vi "PID Fuzzy Control.vi"() -> ()   [LabVIEW 2019]
uses:
  <vilib>/rvi/interface/nirviMethod/nirviMethod.xnode
  <vilib>/FPGAPlugInAG/Dynamic/niLvFpga_Abort_Dynamic.vi
  <vilib>/FPGAPlugInAG/Dynamic/niLvFpga_Run_Dynamic.vi
  <vilib>/rvi/interface/nirviReadWriteControl/nirviReadWriteControl.xnode
  NiFpgaLv.dll
  <vilib>/Utility/error.llb/Error Cluster From Error Code.vi
  <vilib>/rvi/interface/Simulation/niFpgaSimulationCallBeginRW.vi
  <vilib>/rvi/errors/niLvFpgaAdjustHostInterfaceError.vi
  <vilib>/Platform/TimedLoop/XDataNode/wakeup.ctl
  <vilib>/Platform/TimedLoop/XDataNode/XDNodeRunTimeDep.lvlib
  <vilib>/Platform/TimedLoop/XDataNode/nitl_modes.ctl
  <vilib>/Platform/TimedLoop/XDataNode/timing_clust.ctl
  <vilib>/platform/TimedLoop/XDataNode/XDataNode.xnode
  <vilib>/addons/control/pid/NI_PID_pid.lvlib
  <vilib>/addons/control/pid/pid.llb/PID (DBL).vi
  <vilib>/Instr/_visa.llb/VISA Configure Serial Port (Instr).vi
  <vilib>/rvi/interface/nirviOpenFPGA/nirviOpenFPGA.xnode
  <vilib>/addons/Fuzzy Logic/NI_Fuzzy_Logic_API.lvlib
  <vilib>/addons/Fuzzy Logic/FL Fuzzy Controller (SISO).vi
panel:
  out "Numeric":i32
  out "L1 P補償值":dbl
  out "L2 P補償值":dbl
  out "L3 P補償值":dbl
  out "L1 誤差":dbl
  out "L2 誤差":dbl
  out "L3 誤差":dbl
  out "目標角度Chart":cluster{dbl, dbl}[](graph) caption="Waveform Chart - dark"
  in  "VISA resource name":refnum<visa-resource-name>="COM2"
  out "Axis 3比較":cluster{i32[], dbl[]}[](graph)
  out "Axis 2比較":cluster{i32[], dbl[]}[](graph)
  out "Axis 1比較":cluster{i32[], dbl[]}[](graph)
  out "Axis 1":cluster{i32[], dbl[]}(graph)
  out "Axis 3":cluster{i32[], dbl[]}(graph)
  out "Axis 2":cluster{i32[], dbl[]}(graph)
  in  "Period":i64=10
  in  "stop":bool
  out "time loop error":errorcluster
  out "Axis 1 速率 (1mm/s)":dbl
  out "Real Period":u32
  out "沖壓":bool
  out "結束了":bool
  out "Voltage\nOutput":dbl
  out "Voltage\nOutput 2":dbl
  out "Voltage\nOutput 3":dbl
  out "Axis 2 速率 (1mm/s)":dbl
  out "Axis 3 速率 (1mm/s)":dbl
  in  "Axis1 PID gains":T1={"proportional gain (Kc)"=2.0, "integral time (Ti, min)"=0.0, "derivative time (Td, min)"=0.0} {"derivative time (Td, min)" format="%.3f"; "integral time (Ti, min)" format="%.3f"; "proportional gain (Kc)" format="%.3f"}
  in  "Axis 2 PID gains":T1={"proportional gain (Kc)"=2.0, "integral time (Ti, min)"=0.0, "derivative time (Td, min)"=0.0} {"derivative time (Td, min)" format="%.3f"; "integral time (Ti, min)" format="%.3f"; "proportional gain (Kc)" format="%.3f"}
  in  "Axis 3 PID gains":T1={"proportional gain (Kc)"=2.0, "integral time (Ti, min)"=0.0, "derivative time (Td, min)"=0.0} {"derivative time (Td, min)" format="%.3f"; "integral time (Ti, min)" format="%.3f"; "proportional gain (Kc)" format="%.3f"}
  out "實際角度":cluster{"A":dbl, "B":dbl}={"A"=-3.299667554384925, "B"=3.520332445615068}
  out "陀螺儀推算軸長L1":dbl
  out "陀螺儀推算軸長L2":dbl
  out "陀螺儀推算軸長L3":dbl
  out "目標軸長L1":dbl
  out "目標軸長L2":dbl
  out "目標軸長L3":dbl
  out "實際角度Chart":cluster{"X":dbl, "Y":dbl}(graph)={"X"=-3.299667554384925, "Y"=3.520332445615068} caption="Waveform Chart - dark"
  out "目標A":dbl
  out "目標B":dbl
  out "shutdown error":errorcluster
  in  "Tab Control":enum32{"Axis Control"}(tab)
  in  "Axis 1~3 Servo on?":bool
  out "Axis 3 Backward Limit":bool
  out "Axis 3 Backward Limit 2":bool
  out "Axis 2 Backward Limit":bool
  out "Axis 2 Backward Limit 2":bool
  in  "Axis 3 Alarm Reset":bool
  in  "Axis 2 Alarm Reset":bool
  in  "Axis 3 Position Reset":bool
  in  "Axis 2 Position Reset":bool
  in  "Axis 1 Alarm Reset":bool
  in  "Axis 1 Position Reset":bool
  in  "Axis 3 Speed":fxp<+/-,64,32>
  in  "Axis 2 Speed":fxp<+/-,64,32>
  out "Axis 3 Encoder Position (Counts)":i32
  out "Axis 2 Encoder Position (Counts)":i32
  out "Axis 1 Encoder Position (Counts)":i32
  in  "Axis 1 Spped":fxp<+/-,64,32>
  in  "Axis 2 Servo on?":bool
  in  "Axis 3 Servo on?":bool
  in  "Axis 1 Servo on?":bool
  out "Axis 1 Forward Limit":bool
  out "Axis 1 Backward Limit":bool
  out "Timed Out?":bool
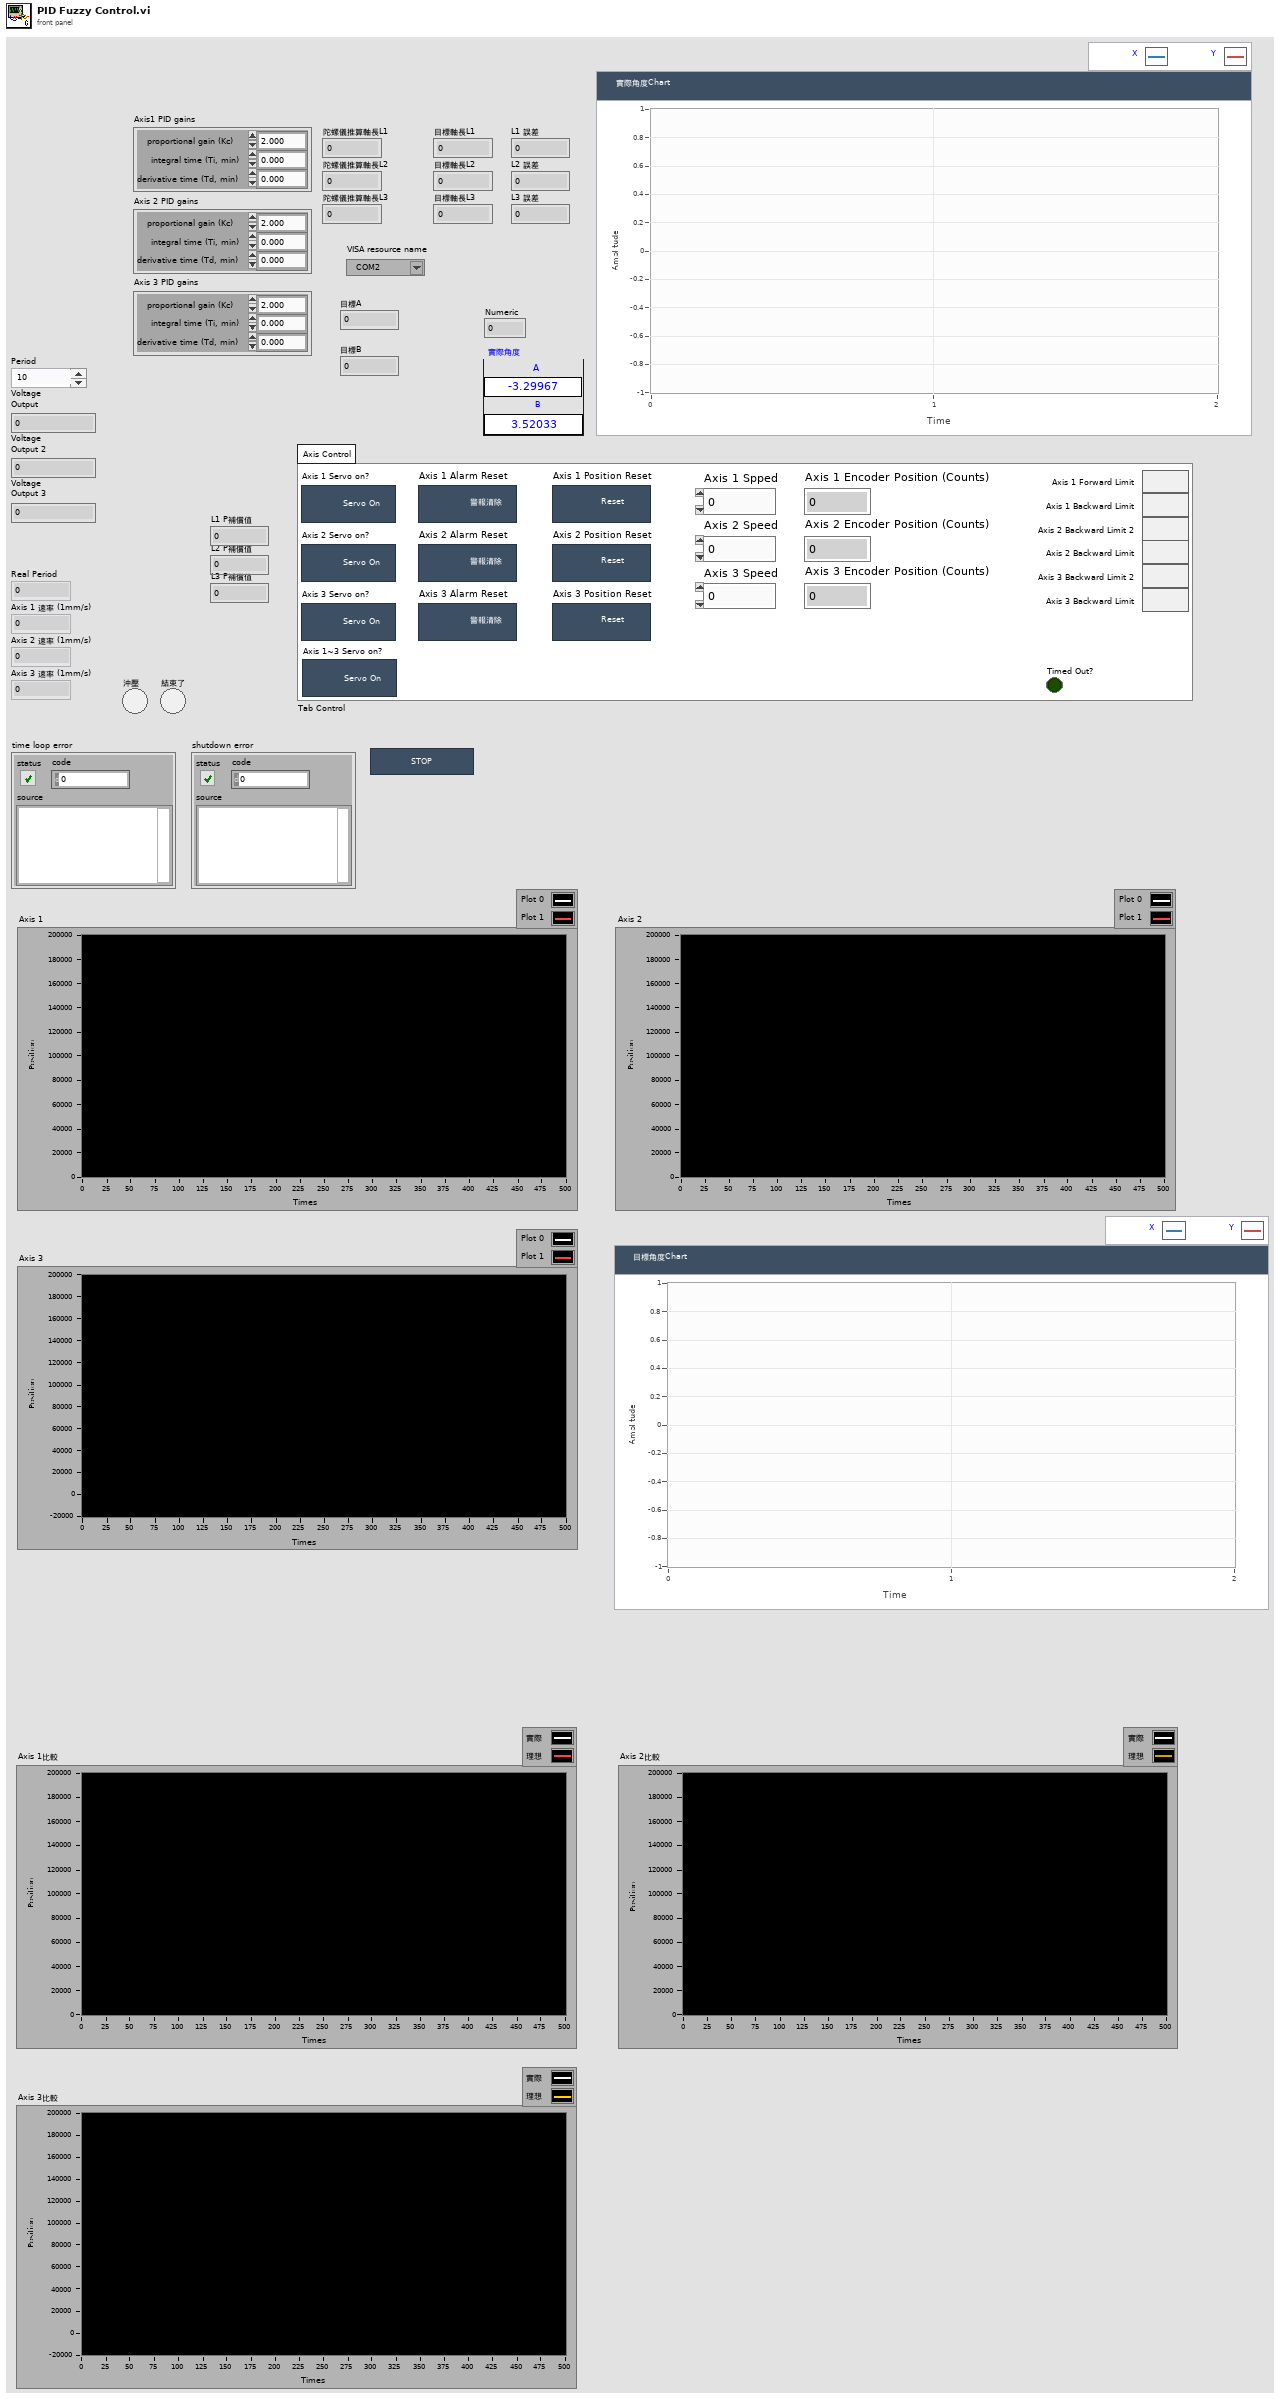
[diagram p1: front panel]
types:
  T1 = cluster{"proportional gain (Kc)":dbl, "integral time (Ti, min)":dbl, "derivative time (Td, min)":dbl}
  T2 = enum16{"open", "replace", "create", "open or create", "replace or create", "replace or create with confirmation"}
  T3 = typedef "XDNodeRunTimeDep.lvlib/timing_clust.ctl" = cluster{"Expected End [f-1]":u64, "Actual End [f-1]":u64, "Finished Late? [f-1]":bool, "Expected End [i-1]":u64, "Actual End [i-1]":u64, "Finished Late? [i-1]":bool, "Expected Start [i]":u64, "Actual Start [i]":u64, "Expected Start [f]":u64, "Actual Start [f]":u64, "Source Name":string, "Structure Name":string, "Period":i64, "Deadline":i64, "Offset":i64, "Start":i64, "Priority":i32, "Timeout":i32, "Mode":T4, "Wakeup Reason":T5, "Error":errorcluster, "Source Type":string, "Secondary Source Type":string, "Global End Time":u64, "Global Start Time":u64, "Frame Duration":u64, "Iteration Duration":u64, "Assigned CPU":i32, "I/O Scan Engine Mode":u32}
  T4 = typedef "XDNodeRunTimeDep.lvlib/nitl_modes.ctl" = enum32{"No Change", "Process missed periods, maintain original phase", "Discard missed periods, maintain original phase", "Process missed periods, ignore original phase", "Discard missed periods, ignore original phase"}
  T5 = typedef "XDNodeRunTimeDep.lvlib/wakeup.ctl" = enum32{"Normal", "Aborted", "Asynchronous wakeup", "Timing source error", "Timed loop error", "Timeout"}
  T6 = typedef "NI_Fuzzy_Logic_API.lvlib/FL System.ctl" = cluster{"input variables":T7[], "output variables":T7[], "rules":T10[], "defuzzification method":T16, "description":string, "user MF interpolating polynomials":T17[]}
  T7 = typedef "NI_Fuzzy_Logic_API.lvlib/FL Variable.ctl" = cluster{"name":string, "range":dbl[], "MFs":T8[]}
  T8 = typedef "NI_Fuzzy_Logic_API.lvlib/FL Membership Function.ctl" = cluster{"name":string, "shape":T9, "points":dbl[], "color":u32, "user-defined shape index":i32}
  T9 = typedef "NI_Fuzzy_Logic_API.lvlib/FL Membership Function Shape.ctl" = u16
  T10 = typedef "NI_Fuzzy_Logic_API.lvlib/FL Rule.ctl" = cluster{"antecedents":T11[], "antecedent connective":T13, "consequents":T14[], "consequent implication":T15, "degree of support":dbl}
  T11 = typedef "NI_Fuzzy_Logic_API.lvlib/FL Antecedent.ctl" = cluster{"Var Index":i32, "MF Index":i32, "Cond":T12}
  T12 = typedef "NI_Fuzzy_Logic_API.lvlib/FL Modifier.ctl" = u16
  T13 = typedef "NI_Fuzzy_Logic_API.lvlib/FL Antecedent Connective.ctl" = u16
  T14 = typedef "NI_Fuzzy_Logic_API.lvlib/FL Consequent.ctl" = cluster{"Var Index":i32, "MF Index":i32, "Cond":T12}
  T15 = typedef "NI_Fuzzy_Logic_API.lvlib/FL Consequent Implication.ctl" = u16
  T16 = typedef "NI_Fuzzy_Logic_API.lvlib/FL Defuzzification.ctl" = u16
  T17 = typedef "NI_Fuzzy_Logic_API.lvlib/FL Interpolating polynomials.ctl" = cluster{"X":dbl[], "Y":dbl[], "Y(x) coeff":dbl[][], "X(y) coeff":dbl[][], "Area(y) coeff":dbl[][], "coa_x(y) coeff":dbl[][]}
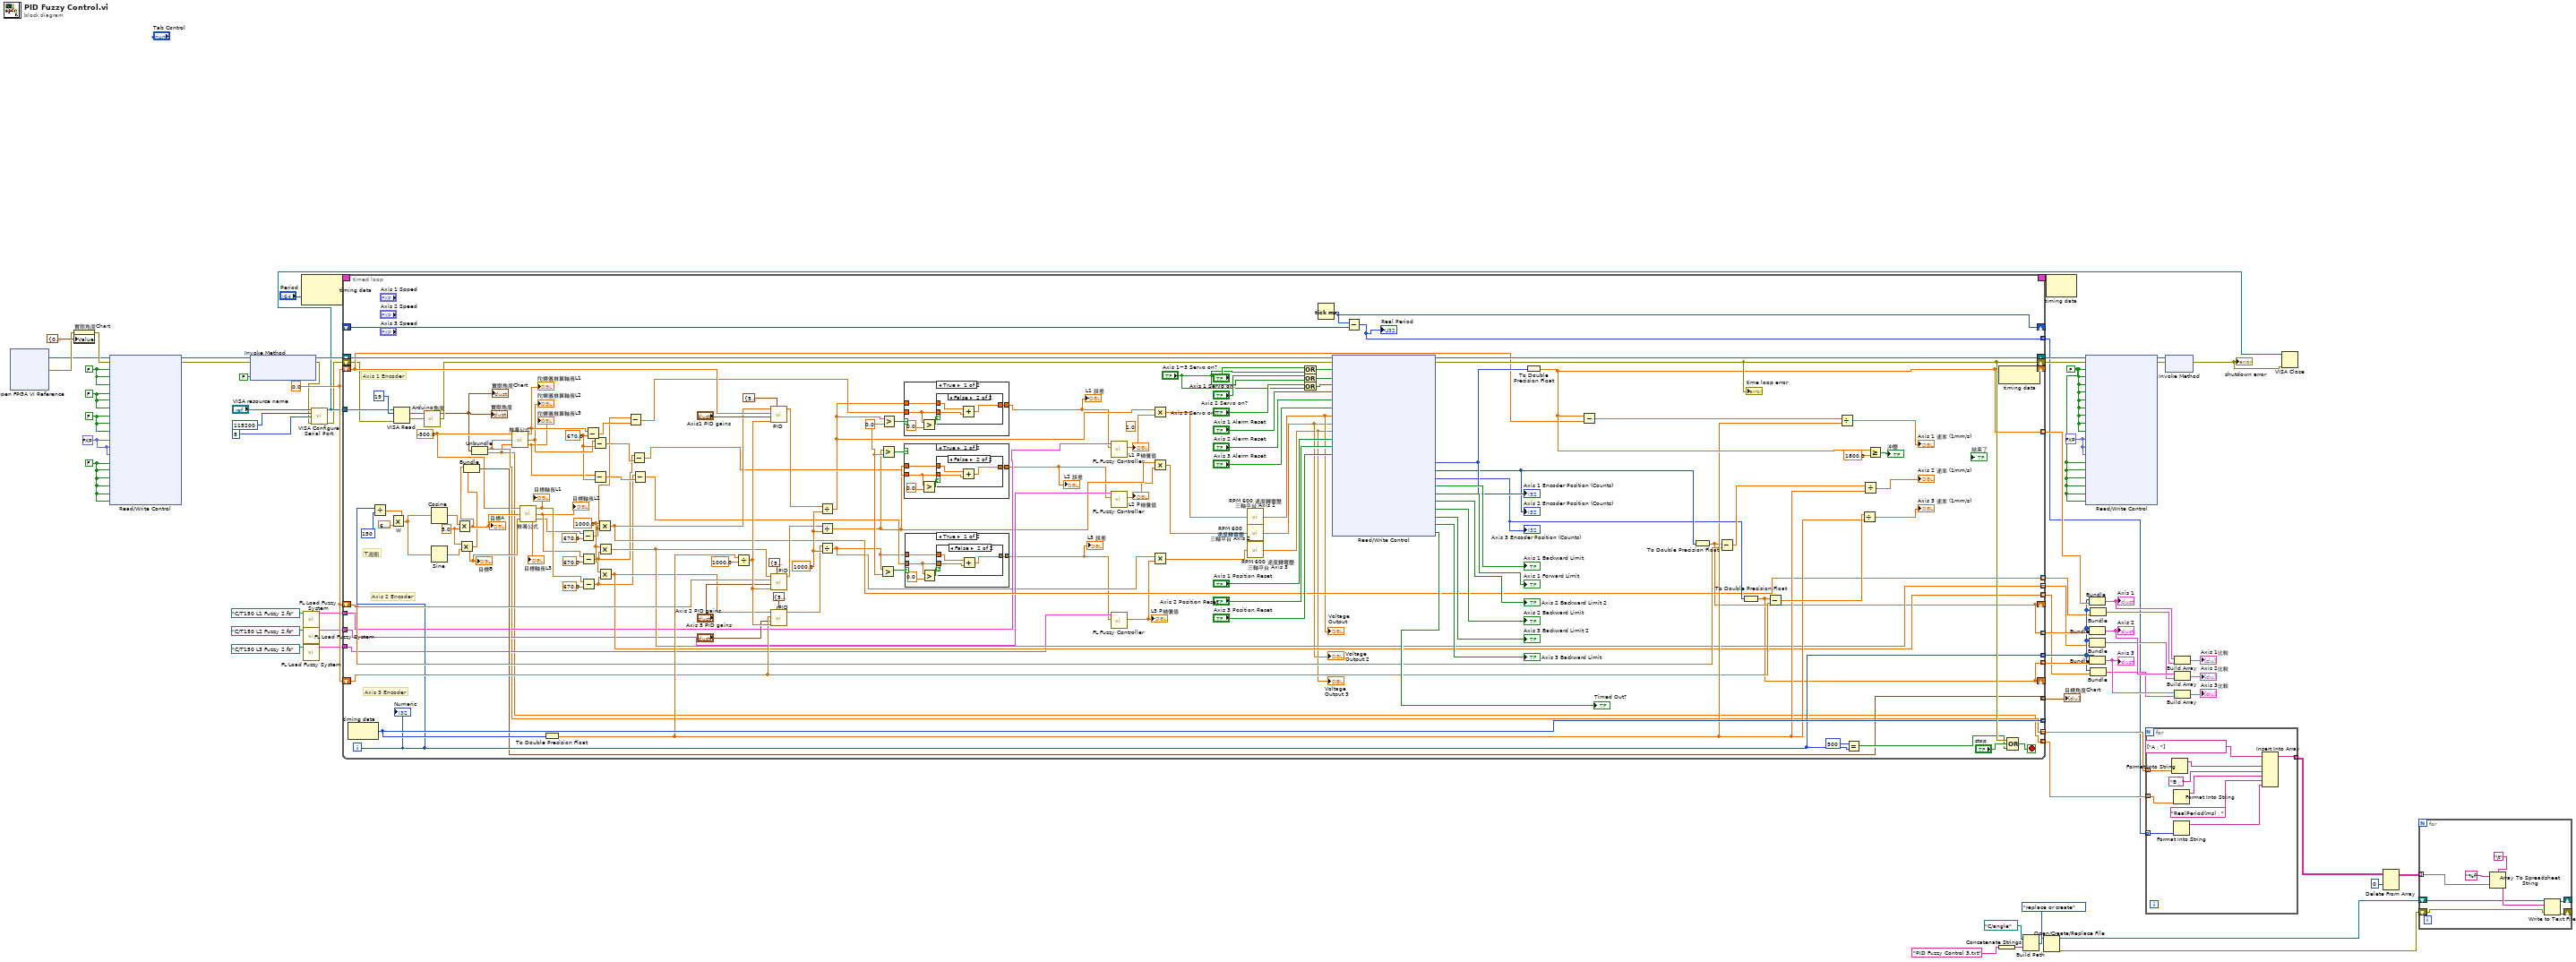
[diagram p0: block diagram]
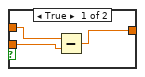
[diagram p2: hidden frame]
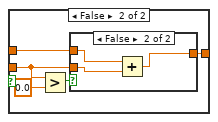
[diagram p3: hidden frame]
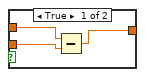
[diagram p4: hidden frame]
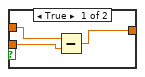
[diagram p5: hidden frame]
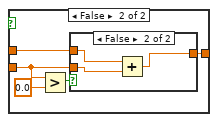
[diagram p6: hidden frame]
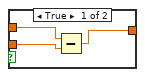
[diagram p7: hidden frame]
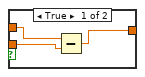
[diagram p8: hidden frame]
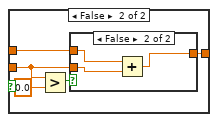
[diagram p9: hidden frame]
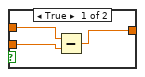
[diagram p10: hidden frame]
diagram:
  w25 = FALSE
  w27 = FALSE
  w52 = 0.0
  w31 = fxp<+,1,1> 0.0
  w30 = FALSE
  w28 = FALSE
  w26 = fxp<+,1,1> 0.0
  w29 = FALSE
  n1 = xnode "Open FPGA VI Reference"() -> ("FPGA VI Reference Out"=w23:refnum<k20>, "error out"=w24:errorcluster)  [unwired: 2 in]
  n2 = property on="實際角度Chart" class="WFChart (strict)"(error in=w24, "Value"=cluster{"X":dbl, "Y":dbl} {"X"=0.0, "Y"=0.0} ("實際角度Chart")) -> (error out=w33:errorcluster)  [unwired: 1 in, 1 out]
  n3 = xnode "Read/Write Control"("FPGA VI Reference In"=w23, "error in"=w33, "Axis 1 Servo on?"=w29, "Axis 2 Servo on?"=w29, "Axis 3 Servo on?"=w29, "Axis 1 Alarm Reset"=w28, "Axis 2 Alarm Reset"=w28, "Axis 3 Alarm Reset"=w28, "Axis 1 Position Reset"=w27, "Axis 2 Position Reset"=w27, "Axis 3 Position Reset"=w27, "Axis 1 Voltage In"=w26, "Axis 2 Voltage In"=w26, "Axis 3 Voltage In"=w26, "Axis 1 Backward Limit"=w25, "Axis 1 Forward Limit"=w25, "Axis 2 Forward Limit"=w25, "Axis 2 Backward Limit"=w25, "Axis 3 ForWard Limit"=w25, "Axis 3 Backward Limit"=w25) -> ("FPGA VI Reference Out"=w64:refnum<k20>, "error out"=w63:errorcluster)
  n4 = xnode "Invoke Method"("FPGA VI Reference In"=w64, "error in"=w63, "Wait Until Done (F)"=FALSE) -> ("FPGA VI Reference Out"=w61:refnum<k20>, "error out"=w22:errorcluster)
  n5 = node-c288("Period") -> (w66:T3)  [unwired: 1 in]
  n6 = call <vilib>:"FL Load Fuzzy System.vi"("file path"=path "C:/T150 L1 Fuzzy 2.fs") -> ("fuzzy system out"=w16:T6)  [unwired: 9 in, 1 out]
  n7 = call <vilib>:"FL Load Fuzzy System.vi"("file path"=path "C:/T150 L2 Fuzzy 2.fs") -> ("fuzzy system out"=w15:T6)  [unwired: 9 in, 1 out]
  n8 = call <vilib>:"FL Load Fuzzy System.vi"("file path"=path "C:/T150 L3 Fuzzy 2.fs") -> ("fuzzy system out"=w14:T6)  [unwired: 9 in, 1 out]
  n9 = call-poly "VISA Configure Serial Port"("VISA resource name"="VISA resource name", "baud rate (9600)"=u32 115200, "data bits (8)"=u16 8, "error in (no error)"=w22) -> ("VISA resource name out"=w40:refnum<visa-resource-name>, "error out"=w21:errorcluster)  [unwired: 10 in]
  n10 = timed-loop {
    shift-right: [w192] -> w57
    shift-left: w61 -> [w191]
    shift-right: [w159] -> w58
    shift-left: w21 -> [w124]
    timing: w66 -> [_]
    timing-out: [_] -> w65
    shift-right: [w154] -> _
    shift-left: w52 -> [w153]
    tunnel: [w158] -> _ mode=indexing
    shift-right: [w188] -> _
    shift-left: _ -> [w189]
    tunnel: [w121] -> w1 mode=indexing
    shift-right: [w113] -> _
    shift-left: w52 -> [w148]
    shift-right: [w112] -> _
    shift-left: w52 -> [w149]
    tunnel: [w129] -> w51 mode=indexing
    tunnel: [w154] -> w55 mode=indexing
    tunnel: [w113] -> w54 mode=indexing
    tunnel: [w112] -> w53 mode=indexing
    tunnel: w40 -> [w125]
    tunnel: [w116] -> w39 mode=indexing
    tunnel: [w115] -> w38 mode=indexing
    tunnel: [w114] -> w37 mode=indexing
    tunnel: [w106] -> w20 mode=indexing
    tunnel: w16 -> [w92]
    tunnel: w15 -> [w91]
    tunnel: w14 -> [w90]
    tunnel: [w82] -> w3 mode=indexing
    tunnel: [w81] -> w2 mode=indexing
    i -> [w129]
    stop <- w190 stop-if-true
    (unwired) 1.0
    w95 = 670.0 ("y")
    w103 = 0.0 ("y")
    w120 = 1000.0 ("x")
    w138 = 5.0 ("y")
    w98 = -500.0 ("移動z")
    w128 = 1000.0 ("x")
    # "T週期"
    # "Axis 3 Encoder"
    # "Axis 2 Encoder"
    # "Axis 1 Encoder"
    n11 = node-c288() -> (w158:i64)  [unwired: 1 in]
    n12 = Divide(x=w129, y=150) -> (x/y=w134:dbl)
    n13 = Multiply "W"(x=w134, y=6.283185307179586) -> (x*y=w133:dbl)
    n14 = VISA Read(VISA resource name=w125, byte count=u32 19, error in (no error)=w124) -> (read buffer=w122:string, error out=w126:errorcluster)  [unwired: 2 out]
    n15 = call "Arduino角度.vi"("error in"=w126, "read buffer"=w122) -> ("error out"=w123:errorcluster, "Waveform Chart"=w70:cluster{dbl, dbl})  [unwired: 1 in, 1 out]
    "實際角度" <- w70
    "實際角度Chart" <- w70
    n16 = Cosine(x=w133) -> (cos(x)=w135:dbl)
    n17 = Sine(x=w133) -> (sin(x)=w136:dbl)
    n18 = Multiply(x=w135, y=w138) -> (x*y=w108:dbl)
    "目標A" <- w108
    n19 = Multiply(x=w138, y=w136) -> (x*y=w107:dbl)
    "目標B" <- w107
    n20 = Bundle(w108, w107) -> (w106:cluster{dbl, dbl})  [unwired: 1 in]
    n21 = Unbundle(w70) -> (w82:dbl, w81:dbl)
    n22 = call "推導公式.vi"("be"=w81, "al"=w82, "移動z"=w98) -> ("L3"=w80:dbl, "L2"=w96:dbl, "L1"=w97:dbl)
    "陀螺儀推算軸長L1" <- w97
    "陀螺儀推算軸長L2" <- w96
    "陀螺儀推算軸長L3" <- w80
    n23 = call "推導公式.vi"("be"=w107, "al"=w108, "移動z"=w98) -> ("L3"=w99:dbl, "L2"=w100:dbl, "L1"=w101:dbl)
    "目標軸長L1" <- w101
    "目標軸長L2" <- w100
    "目標軸長L3" <- w99
    n24 = To Double Precision Float(number=w158) -> (double precision float=w151:dbl)
    n25 = Subtract(x=w99, y=670.0) -> (x-y=w83:dbl)
    n26 = Subtract(x=w100, y=670.0) -> (x-y=w85:dbl)
    n27 = Subtract(x=w101, y=670.0) -> (x-y=w88:dbl)
    n28 = Subtract(x=w97, y=w95) -> (x-y=w93:dbl)
    n29 = Subtract(x=w96, y=w95) -> (x-y=w86:dbl)
    n30 = Subtract(x=w80, y=w95) -> (x-y=w94:dbl)
    n31 = Multiply(x=w128, y=w83) -> (x*y=w116:dbl)
    n32 = Multiply(x=w128, y=w85) -> (x*y=w115:dbl)
    n33 = Multiply(x=w128, y=w88) -> (x*y=w114:dbl)
    n34 = Subtract(x=w83, y=w93) -> (x-y=w84:dbl)
    n35 = Subtract(x=w85, y=w86) -> (x-y=w87:dbl)
    n36 = Subtract(x=w88, y=w94) -> (x-y=w89:dbl)
    n37 = Divide(x=w151, y=1000.0) -> (x/y=w150:dbl)
    n38 = call-poly <vilib>:"PID.vi"("output range"=cluster{"output high":dbl, "output low":dbl} {"output high"=50000.0, "output low"=-50000.0}, "dt (s)"=w150, "PID gains"="Axis1 PID gains", "process variable"=w153, "setpoint"=w116) -> ("output"=w119:dbl)  [unwired: 5 in, 1 out]
    n39 = call-poly <vilib>:"PID.vi"("output range"=cluster{"output high":dbl, "output low":dbl} {"output high"=50000.0, "output low"=-50000.0}, "dt (s)"=w150, "PID gains"="Axis 2 PID gains", "process variable"=w148, "setpoint"=w115) -> ("output"=w118:dbl)  [unwired: 5 in, 1 out]
    n40 = call-poly <vilib>:"PID.vi"("output range"=cluster{"output high":dbl, "output low":dbl} {"output high"=50000.0, "output low"=-50000.0}, "dt (s)"=w150, "PID gains"="Axis 3 PID gains", "process variable"=w149, "setpoint"=w114) -> ("output"=w117:dbl)  [unwired: 5 in, 1 out]
    n41 = Divide(x=w119, y=w120) -> (x/y=w76:dbl)
    n42 = Divide(x=w118, y=w120) -> (x/y=w74:dbl)
    n43 = Divide(x=w117, y=w120) -> (x/y=w79:dbl)
    n44 = Greater?(x=w79, y=w103) -> (0:w102:bool)
    n45 = Greater?(x=w74, y=w103) -> (0:w104:bool)
    n46 = Greater?(x=w76, y=w103) -> (0:w105:bool)
    n47 = case shown="True" w105 {
      tunnel: [w240 w251] -> w73
      tunnel: w84 -> [w238 w249]
      tunnel: w76 -> [w239 w250]
      frame True {
        n48 = Greater?(x=w238, y=0.0) -> (0:w241:bool)
        n49 = case shown="False" w241 {
          tunnel: [w245 w248] -> w240
          tunnel: w239 -> [w244 w247]
          tunnel: w238 -> [w243 w246]
          frame True {
            n50 = Subtract(x=w244, y=w243) -> (x-y=w245:dbl)
          }
          frame False {
            n51 = Add(x=w247, y=w246) -> (x+y=w248:dbl)
          }
        }
      }
      frame False {
        n52 = Greater?(x=w249, y=0.0) -> (0:w252:bool)
        n53 = case shown="False" w252 {
          tunnel: [w256 w259] -> w251
          tunnel: w250 -> [w255 w258]
          tunnel: w249 -> [w254 w257]
          frame True {
            n54 = Subtract(x=w255, y=w254) -> (x-y=w256:dbl)
          }
          frame False {
            n55 = Add(x=w258, y=w257) -> (x+y=w259:dbl)
          }
        }
      }
    }
    "L1 誤差" <- w73
    n56 = case shown="True" w104 {
      tunnel: [w218 w229] -> w72
      tunnel: w87 -> [w216 w227]
      tunnel: w74 -> [w217 w228]
      frame True {
        n57 = Greater?(x=w216, y=0.0) -> (0:w219:bool)
        n58 = case shown="False" w219 {
          tunnel: [w223 w226] -> w218
          tunnel: w217 -> [w222 w225]
          tunnel: w216 -> [w221 w224]
          frame True {
            n59 = Subtract(x=w222, y=w221) -> (x-y=w223:dbl)
          }
          frame False {
            n60 = Add(x=w225, y=w224) -> (x+y=w226:dbl)
          }
        }
      }
      frame False {
        n61 = Greater?(x=w227, y=0.0) -> (0:w230:bool)
        n62 = case shown="False" w230 {
          tunnel: [w234 w237] -> w229
          tunnel: w228 -> [w233 w236]
          tunnel: w227 -> [w232 w235]
          frame True {
            n63 = Subtract(x=w233, y=w232) -> (x-y=w234:dbl)
          }
          frame False {
            n64 = Add(x=w236, y=w235) -> (x+y=w237:dbl)
          }
        }
      }
    }
    "L2 誤差" <- w72
    n65 = case shown="True" w102 {
      tunnel: [w196 w207] -> w71
      tunnel: w89 -> [w194 w205]
      tunnel: w79 -> [w195 w206]
      frame True {
        n66 = Greater?(x=w194, y=0.0) -> (0:w197:bool)
        n67 = case shown="False" w197 {
          tunnel: [w201 w204] -> w196
          tunnel: w195 -> [w200 w203]
          tunnel: w194 -> [w199 w202]
          frame True {
            n68 = Subtract(x=w200, y=w199) -> (x-y=w201:dbl)
          }
          frame False {
            n69 = Add(x=w203, y=w202) -> (x+y=w204:dbl)
          }
        }
      }
      frame False {
        n70 = Greater?(x=w205, y=0.0) -> (0:w208:bool)
        n71 = case shown="False" w208 {
          tunnel: [w212 w215] -> w207
          tunnel: w206 -> [w211 w214]
          tunnel: w205 -> [w210 w213]
          frame True {
            n72 = Subtract(x=w211, y=w210) -> (x-y=w212:dbl)
          }
          frame False {
            n73 = Add(x=w214, y=w213) -> (x+y=w215:dbl)
          }
        }
      }
    }
    "L3 誤差" <- w71
    n74 = call-poly <vilib>:"FL Fuzzy Controller.vi"("input value"=w73, "fuzzy system in"=w92) -> ("output value"=w69:dbl)  [unwired: 5 in, 4 out]
    "L1 P補償值" <- w69
    n75 = call-poly <vilib>:"FL Fuzzy Controller.vi"("input value"=w72, "fuzzy system in"=w91) -> ("output value"=w68:dbl)  [unwired: 5 in, 4 out]
    "L2 P補償值" <- w68
    n76 = call-poly <vilib>:"FL Fuzzy Controller.vi"("input value"=w71, "fuzzy system in"=w90) -> ("output value"=w67:dbl)  [unwired: 5 in, 4 out]
    "L3 P補償值" <- w67
    n77 = Multiply(x=w76, y=w69) -> (x*y=w75:dbl)
    n78 = Multiply(x=w74, y=w68) -> (x*y=w77:dbl)
    n79 = Multiply(x=w79, y=w67) -> (x*y=w78:dbl)
    n80 = call "RPM 600 速度轉電壓 三軸平台 Axis 1.vi"("Speed (1mm/s)"=w75) -> ("Voltage\nOutput"=w111:dbl)
    "Voltage\nOutput" <- w111
    n81 = call "RPM 600 速度轉電壓 三軸平台 Axis 2.vi"("Speed (1mm/s)"=w77) -> ("Voltage\nOutput"=w110:dbl)
    "Voltage\nOutput 2" <- w110
    n82 = call "RPM 600 速度轉電壓 三軸平台 Axis 3.vi"("Speed (1mm/s)"=w78) -> ("Voltage\nOutput"=w109:dbl)
    "Voltage\nOutput 3" <- w109
    n83 = Or(x="Axis 1 Servo on?", y="Axis 1~3 Servo on?") -> (x .or. y?=w171:bool)
    n84 = Or(x="Axis 2 Servo on?", y="Axis 1~3 Servo on?") -> (x .or. y?=w168:bool)
    n85 = Or(x="Axis 3 Servo on?", y="Axis 1~3 Servo on?") -> (x .or. y?=w166:bool)
    n86 = Tick Count (ms)() -> (millisecond timer value=w188:u32)
    n87 = xnode "Read/Write Control"("FPGA VI Reference In"=w191, "error in"=w123, "Axis 1 Servo on?"=w171, "Axis 2 Servo on?"=w168, "Axis 3 Servo on?"=w166, "Axis 1 Alarm Reset"="Axis 1 Alarm Reset", "Axis 2 Alarm Reset"="Axis 2 Alarm Reset", "Axis 3 Alarm Reset"="Axis 3 Alarm Reset", "Axis 1 Voltage In"=w111, "Axis 2 Voltage In"=w110, "Axis 3 Voltage In"=w109, "Axis 1 Position Reset"="Axis 1 Position Reset", "Axis 2 Position Reset"="Axis 2 Position Reset", "Axis 3 Position Reset"="Axis 3 Position Reset") -> ("FPGA VI Reference Out"=w192:refnum<k20>, "error out"=w159:errorcluster, "Axis 1 Encoder Position (Counts)"=w164:i32, "Axis 2 Encoder Position (Counts)"=w162:i32, "Axis 3 Encoder Position (Counts)"=w161:i32, "Axis 1 Backward Limit"=→"Axis 1 Backward Limit":bool, "Axis 1 Forward Limit"=→"Axis 1 Forward Limit":bool, "Axis 2 Backward Limit"=→"Axis 2 Backward Limit 2":bool, "Axis 2 Forward Limit"=→"Axis 2 Backward Limit":bool, "Axis 3 Backward Limit"=→"Axis 3 Backward Limit 2":bool, "Axis 3 ForWard Limit"=→"Axis 3 Backward Limit":bool, "Timed Out?"=→"Timed Out?":bool)
    "time loop error" <- w159
    "Axis 1 Encoder Position (Counts)" <- w164
    "Axis 2 Encoder Position (Counts)" <- w162
    "Axis 3 Encoder Position (Counts)" <- w161
    n88 = Subtract(x=w188, y=w189) -> (x-y=w121:u32)
    "Real Period" <- w121
    n89 = To Double Precision Float(number=w164) -> (double precision float=w154:dbl)
    n90 = Subtract(x=w154, y=w153) -> (x-y=w193:dbl)
    n91 = To Double Precision Float(number=w162) -> (double precision float=w113:dbl)
    n92 = Subtract(x=w113, y=w148) -> (x-y=w163:dbl)
    n93 = To Double Precision Float(number=w161) -> (double precision float=w112:dbl)
    n94 = Subtract(x=w112, y=w149) -> (x-y=w160:dbl)
    n95 = Divide(x=w193, y=w151) -> (x/y=→"Axis 1 速率 (1mm/s)":dbl)
    n96 = Equal?(x=500, y=w129) -> (x = y?=w140:bool)
    n97 = Divide(x=w160, y=w151) -> (x/y=→"Axis 3 速率 (1mm/s)":dbl)
    n98 = Divide(x=w163, y=w151) -> (x/y=→"Axis 2 速率 (1mm/s)":dbl)
    n99 = Greater Or Equal?(x=w154, y=1800.0) -> (x >= y?=→"沖壓":bool)
    n100 = node-c288() -> ()  [unwired: 1 in, 1 out]
    n101 = Compound Arithmetic op=OR(w159, "stop", w140) -> (w190:bool)
    "Numeric" <- w129
  }
  "目標角度Chart" <- w20
  n102 = Concatenate Strings("PID Fuzzy Control 3.txt" ("element")) -> (w12:string)
  n103 = Build Path(base path=path "C:/angle", name or relative path=w12) -> (appended path=w13:path)
  n104 = Open/Create/Replace File(file path (use dialog)=w13, operation (0:open)=T2."replace or create") -> (refnum out=w6:refnum<file>, error out=w5:errorcluster)  [unwired: 4 in, 1 out]
  n105 = node-c288(w65) -> ()  [unwired: 1 out]
  n106 = xnode "Read/Write Control"("FPGA VI Reference In"=w57, "error in"=w58, "Axis 1 Servo on?"=w30, "Axis 2 Servo on?"=w30, "Axis 3 Servo on?"=w30, "Axis 1 Alarm Reset"=w30, "Axis 2 Alarm Reset"=w30, "Axis 3 Alarm Reset"=w30, "Axis 1 Position Reset"=w30, "Axis 2 Position Reset"=w30, "Axis 3 Position Reset"=w30, "Axis 1 Voltage In"=w31, "Axis 2 Voltage In"=w31, "Axis 3 Voltage In"=w31, "Axis 1 Backward Limit"=w30, "Axis 1 Forward Limit"=w30, "Axis 2 Forward Limit"=w30, "Axis 2 Backward Limit"=w30, "Axis 3 ForWard Limit"=w30, "Axis 3 Backward Limit"=w30) -> ("FPGA VI Reference Out"=w60:refnum<k20>, "error out"=w59:errorcluster)
  n107 = Bundle(w51, w55) -> (w50:cluster{i32[], dbl[]})  [unwired: 1 in]
  "Axis 1" <- w50
  n108 = Bundle(w51, w54) -> (w49:cluster{i32[], dbl[]})  [unwired: 1 in]
  "Axis 2" <- w49
  n109 = Bundle(w51, w38) -> (w35:cluster{i32[], dbl[]})  [unwired: 1 in]
  n110 = Bundle(w51, w53) -> (w48:cluster{i32[], dbl[]})  [unwired: 1 in]
  "Axis 3" <- w48
  n111 = Bundle(w51, w39) -> (w36:cluster{i32[], dbl[]})  [unwired: 1 in]
  n112 = Bundle(w51, w37) -> (w34:cluster{i32[], dbl[]})  [unwired: 1 in]
  n113 = for {
    tunnel: [w270] -> w4 mode=indexing
    tunnel: w3 -> [w265] mode=indexing
    tunnel: w2 -> [w264] mode=indexing
    tunnel: w1 -> [w263] mode=indexing
    n114 = Format Into String(w265) -> (resulting string=w267:string)  [unwired: 3 in, 1 out]
    n115 = Format Into String(w264) -> (resulting string=w268:string)  [unwired: 3 in, 1 out]
    n116 = Format Into String(w263) -> (resulting string=w269:string)  [unwired: 3 in, 1 out]
    n117 = Insert Into Array(array=string[] ["A："], new element #1=w267, new element #2="B：", new element #3=w268, new element #4="RealPeriod(ms)：", new element #5=w269) -> (w270:string[])  [unwired: 1 in]
  }
  n118 = xnode "Invoke Method"("FPGA VI Reference In"=w60, "error in"=w59) -> ("error out"=w41:errorcluster)  [unwired: 1 out]
  "shutdown error" <- w41
  n119 = Build Array(w50, w36) -> (→"Axis 1比較":cluster{i32[], dbl[]}[])
  n120 = Build Array(w49, w35) -> (→"Axis 2比較":cluster{i32[], dbl[]}[])
  n121 = Build Array(w48, w34) -> (→"Axis 3比較":cluster{i32[], dbl[]}[])
  n122 = VISA Close(VISA resource name=w40, error in (no error)=w41) -> ()  [unwired: 1 out]
  n123 = Delete From Array(array=w4, index (row)=0) -> (array with subset deleted=w8:string[][])  [unwired: 2 in, 1 out]
  n124 = for {
    shift-right: [w274] -> _
    shift-left: w6 -> [w277]
    shift-right: [w275] -> _
    shift-left: w5 -> [w276]
    tunnel: w8 -> [w273] mode=indexing
    n125 = Array To Spreadsheet String(delimiter (Tab)="\t", array=w273, 3:"%f" ("format string")) -> (spreadsheet string=w278:string)
    n126 = Write to Text File(file (use dialog)=w277, text=w278, error in=w276) -> (refnum out=w274:refnum<file>, error out=w275:errorcluster)  [unwired: 1 in, 1 out]
  }
